vi "PPMS_Femto_SetAll.vi"(8 "4 - control":T1={"3 - Gain_1 i"=FALSE, "3 - Gain_2 i"=FALSE, "3 - AC/DC"=TRUE, "3 - Filter"=TRUE}, 9 "3 - control":T1={"3 - Gain_1 i"=FALSE, "3 - Gain_2 i"=FALSE, "3 - AC/DC"=TRUE, "3 - Filter"=TRUE}, 10 "2 - Gain Exponent (10^  A/V)":dbl(slide)=4.0 min=4.0 max=13.0 step=1.0 scale=4.0..13.0, 11 "1 - Gain Exponent (10^  A/V)":dbl(slide)=4.0 min=4.0 max=13.0 step=1.0 scale=4.0..13.0) -> ()   [LabVIEW 2013]
uses:
  driver/FEMTO_LUCI-10.lvlib
panel:
  out "4 - Gain_Stages":bool[](array[boolean])=[FALSE, FALSE, FALSE, TRUE, FALSE, FALSE, FALSE, FALSE, FALSE, FALSE, FALSE, FALSE, FALSE, FALSE, FALSE, FALSE, FALSE, FALSE, FALSE, FALSE, FALSE, FALSE, FALSE, FALSE, FALSE, FALSE, FALSE, FALSE, FALSE, FALSE, FALSE, FALSE]
  out "4 - Overload":bool
  out "3 - Overload":bool
  out "3 - Gain_Stages 2":bool[](array[boolean])=[FALSE, FALSE, FALSE, TRUE, FALSE, FALSE, FALSE, FALSE, FALSE, FALSE, FALSE, FALSE, FALSE, FALSE, FALSE, FALSE, FALSE, FALSE, FALSE, FALSE, FALSE, FALSE, FALSE, FALSE, FALSE, FALSE, FALSE, FALSE, FALSE, FALSE, FALSE, FALSE]
  out "2 - Overload":bool
  out "1 - Overload":bool
  # "1"
  # "2"
  # "3"
  # "4"
  # "80 dB"
  # "60 dB"
  # "40 dB"
  # "20 dB"
  # "1 kHz"
  # "100 kHz"
  # "AC"
  # "DC"
  # "20 dB"
  # "40 dB"
  # "0 dB"
  # "0 dB"
  # "1 kHz"
  # "100 kHz"
  # "AC"
  # "DC"
  # "20 dB"
  # "40 dB"
  # "0 dB"
  # "0 dB"
  # "80 dB"
  # "60 dB"
  # "40 dB"
  # "20 dB"
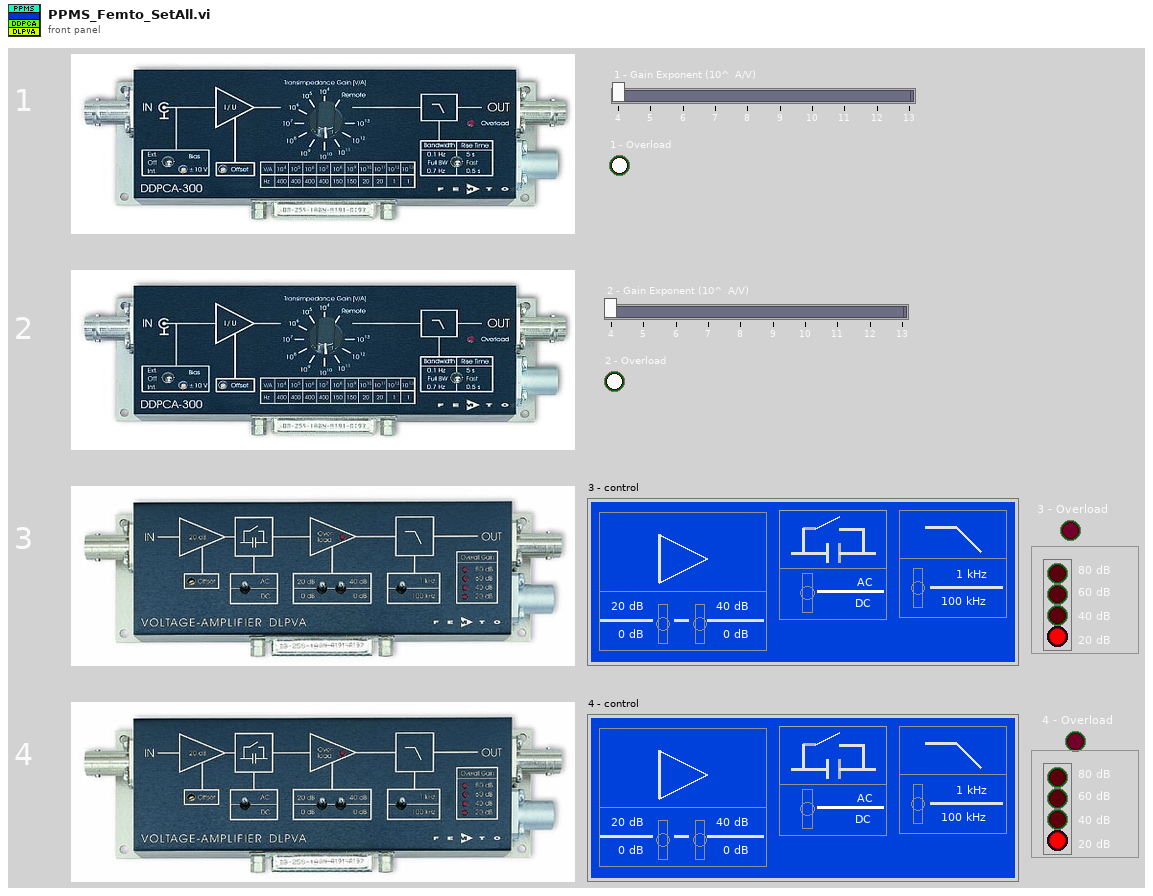
[diagram p1: front panel]
types:
  T1 = cluster{"3 - Gain_1 i":bool, "3 - Gain_2 i":bool, "3 - AC/DC":bool, "3 - Filter":bool}
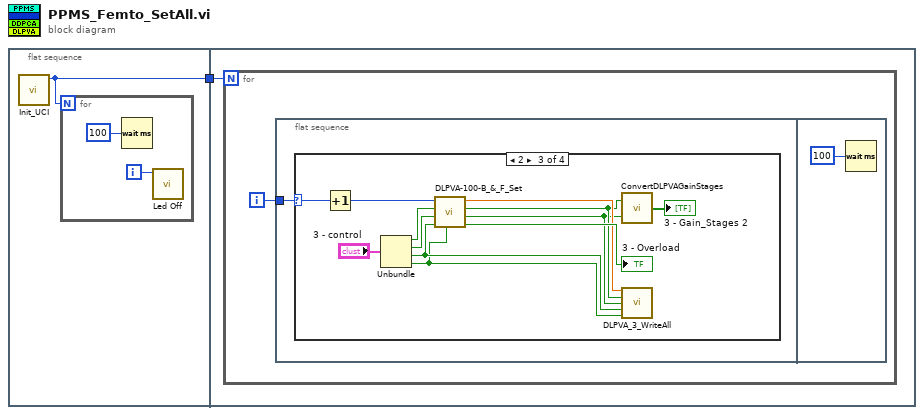
[diagram p0: block diagram]
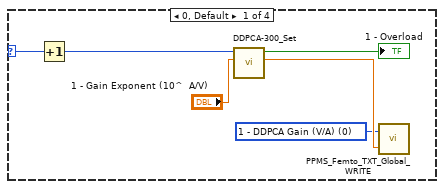
[diagram p2: hidden frame]
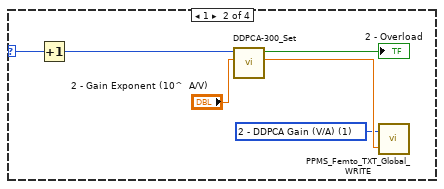
[diagram p3: hidden frame]
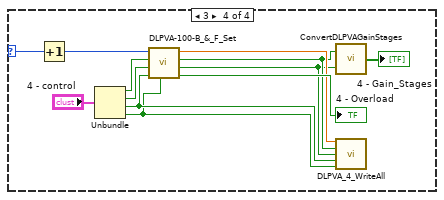
[diagram p4: hidden frame]
diagram:
  n1 = flat-sequence {
    tunnel: [w2] -> w1
    tunnel: w1 -> [w5]
    frame #0 {
      n2 = call "Init_UCI.vi"() -> ("Number of Devices"=w2:i32)  [unwired: 10 in, 1 out]
      n3 = for {
        N: w2 -> [_]
        i -> [w4]
        n4 = Wait (ms)(milliseconds to wait=u32 100) -> ()  [unwired: 1 out]
        n5 = call "Led Off.vi"("index"=w4) -> ()  [unwired: 9 in, 2 out]
      }
    }
    frame #1 {
      n6 = for {
        N: w5 -> [_]
        i -> [w6]
        n7 = flat-sequence {
          tunnel: w6 -> [w7]
          frame #0 {
            n8 = case shown="2" w7 {
              selector: w7 -> [w11 w19 w31 w43]
              frame 0, Default {
                w8 = u16 0 items=["1 - DDPCA Gain (V/A)", "2 - DDPCA Gain (V/A)", "3 - DLPVA Gain (dB)", "3 - Gain 1", "3 - Gain 2", "3 - AC/DC coupling", "3 - filter", "4 - DLPVA Gain (dB)", "4 - Gain 1", "4 - Gain 2", "4 - AC/DC coupling", "4 - filter"] ("Property")
                n9 = Increment(x=w11) -> (x+1=w10:i32)
                n10 = call "DDPCA-300_Set.vi"("Gain Exponent (10^  A/V)"="1 - Gain Exponent (10^  A/V)", "Index"=w10) -> ("Gain (V/A)"=w9:dbl, "Overload"=→"1 - Overload":bool)  [unwired: 8 in]
                n11 = call "PPMS_Femto_TXT_Global_WRITE.vi"("Value"=w9, "Property"=w8) -> ()  [unwired: 2 in]
              }
              frame 1 {
                w14 = u16 1 items=["1 - DDPCA Gain (V/A)", "2 - DDPCA Gain (V/A)", "3 - DLPVA Gain (dB)", "3 - Gain 1", "3 - Gain 2", "3 - AC/DC coupling", "3 - filter", "4 - DLPVA Gain (dB)", "4 - Gain 1", "4 - Gain 2", "4 - AC/DC coupling", "4 - filter"] ("Property")
                n12 = Increment(x=w19) -> (x+1=w16:i32)
                n13 = call "DDPCA-300_Set.vi"("Gain Exponent (10^  A/V)"="2 - Gain Exponent (10^  A/V)", "Index"=w16) -> ("Gain (V/A)"=w15:dbl, "Overload"=→"2 - Overload":bool)  [unwired: 8 in]
                n14 = call "PPMS_Femto_TXT_Global_WRITE.vi"("Value"=w15, "Property"=w14) -> ()  [unwired: 2 in]
              }
              frame 2 {
                n15 = Increment(x=w31) -> (x+1=w29:i32)
                n16 = Unbundle("3 - control") -> ("3 - Gain_1 i"=w27:bool, "3 - Gain_2 i"=w26:bool, "3 - AC/DC"=w21:bool, "3 - Filter"=w20:bool)
                n17 = call "DLPVA-100-B_&_F_Set.vi"("Filter"=w20, "AC/DC"=w21, "Gain_2 i"=w26, "Gain_1 i"=w27, "Index"=w29) -> ("Overload"=→"3 - Overload":bool, "Gain_2 o"=w22:bool, "Gain_1o"=w23:bool, "Gain (dB)"=w24:dbl)  [unwired: 3 in]
                n18 = call "ConvertDLPVAGainStages.vi"("Gain_2 i"=w22, "Gain_1 i"=w23) -> ("Array"=→"3 - Gain_Stages 2":bool[])
                n19 = call "DLPVA_3_WriteAll.vi"("Gain (dB)"=w24, "Gain_1o"=w23, "Gain_2 o"=w22, "AC/DC o"=w21, "Filter o"=w20) -> ()  [unwired: 11 in]
              }
              frame 3 {
                n20 = Increment(x=w43) -> (x+1=w42:i32)
                n21 = Unbundle("4 - control") -> ("3 - Gain_1 i"=w40:bool, "3 - Gain_2 i"=w39:bool, "3 - AC/DC"=w33:bool, "3 - Filter"=w32:bool)
                n22 = call "DLPVA-100-B_&_F_Set.vi"("Filter"=w32, "AC/DC"=w33, "Gain_2 i"=w39, "Gain_1 i"=w40, "Index"=w42) -> ("Overload"=→"4 - Overload":bool, "Gain_2 o"=w34:bool, "Gain_1o"=w35:bool, "Gain (dB)"=w36:dbl)  [unwired: 3 in]
                n23 = call "ConvertDLPVAGainStages.vi"("Gain_2 i"=w34, "Gain_1 i"=w35) -> ("Array"=→"4 - Gain_Stages":bool[])
                n24 = call "DLPVA_4_WriteAll.vi"("Gain (dB)"=w36, "Gain_1o"=w35, "Gain_2 o"=w34, "AC/DC o"=w33, "Filter o"=w32) -> ()  [unwired: 11 in]
              }
            }
          }
          frame #1 {
            n25 = Wait (ms)(milliseconds to wait=u32 100) -> ()  [unwired: 1 out]
          }
        }
      }
    }
  }
